vi "Tresorie_nette.vi"(1 "Dettes":dbl, 2 "Argent ventes":dbl) -> (0 "tresorire nette":dbl)   [LabVIEW 2024]
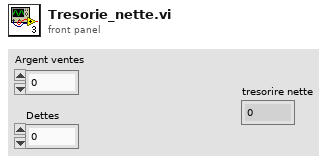
[diagram p1: front panel]
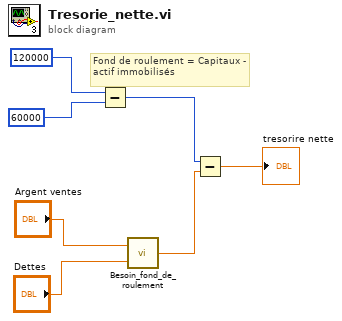
[diagram p0: block diagram]
diagram:
  # "Fond de roulement = Capitaux - actif immobilisés"
  n1 = Subtract(x=120000, y=60000) -> (x-y=w3:i32)
  n2 = call "Besoin_fond_de_roulement.vi"("Argent ventes"="Dettes", "dettes"="Argent ventes") -> ("BFR"=w2:dbl)
  n3 = Subtract(x=w3, y=w2) -> (x-y=→"tresorire nette":dbl)
